vi "Process.vi"(8 "error in (no error)":errorcluster, 9 "New polarization":dbl, 10 "New eventnum":i64, 11 "Automation in":refnum<class "NMR Data.lvclass">) -> (0 "error out":errorcluster, 2 "Added new data point?":bool, 3 "Automation out":refnum<class "NMR Data.lvclass">)   [LabVIEW 2019, in "NMR Data.lvclass"]
uses:
  NMR Data.lvclass
  NMR Data.lvclass/NMR Data.ctl
panel:
  out "Eventnums":i64[](array[numeric])
  out "Polarizations":dbl[](array[numeric])
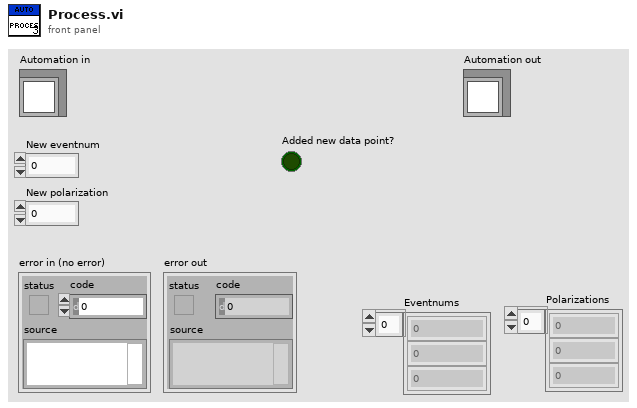
[diagram p1: front panel]
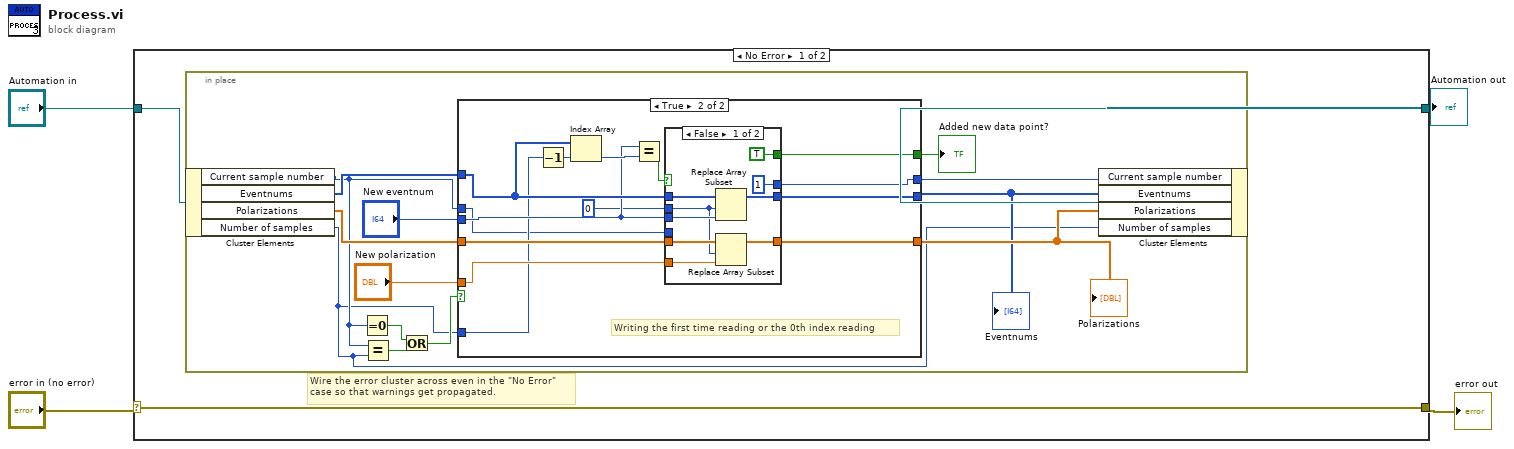
[diagram p0: block diagram]
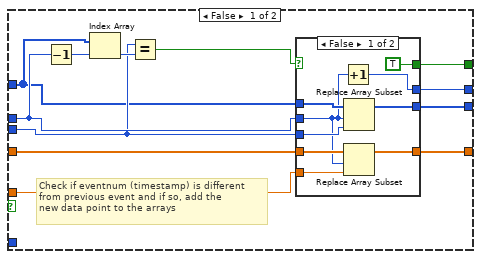
[diagram p2: hidden frame]
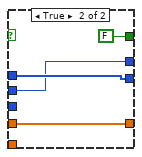
[diagram p3: hidden frame]
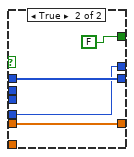
[diagram p4: hidden frame]
diagram:
  n1 = case shown="No Error" "error in (no error)" {
    selector: "error in (no error)" -> [w7 w74]
    tunnel: [w7 w74] -> w3
    tunnel: [w5 w73] -> w1
    tunnel: "Automation in" -> [w6 w73]
    frame No Error {
      # "Wire the error cluster across even in the \"No Error\"\ncase so that warnings get propagated."
      n2 = in-place {
        n3 = in-place-cluster #1(w6) -> ("Current sample number"=w12:i32, "Eventnums"=w17:i64[], "Polarizations"=w16:dbl[], "Number of samples"=w8:i32)
        n4 = Equal To 0?(x=w12) -> (x = 0?=w10:bool)
        n5 = Equal?(x=w12, y=w8) -> (x = y?=w11:bool)
        n6 = Or(x=w10, y=w11) -> (x .or. y?=w9:bool)
        n7 = case shown="True" w9 {
          tunnel: w12 -> [w29 w46]
          tunnel: [w21 w49] -> w13
          tunnel: "New eventnum" -> [w27 w52]
          tunnel: w17 -> [w25 w53]
          tunnel: w16 -> [w28 w59]
          tunnel: "New polarization" -> [w26 w58]
          tunnel: [w22 w57] -> w14
          tunnel: [w23 w56] -> w15
          tunnel: [w24 w47] -> w18
          tunnel: w8 -> [_ w48]
          frame False {
            # "Check if eventnum (timestamp) is different\nfrom previous event and if so, add the\nnew data point to the arrays"
            n8 = Decrement(x=w29) -> (x-1=w30:i32)
            n9 = Index Array(array=w25, index=w30) -> (element=w31:i64)
            n10 = Equal?(x=w27, y=w31) -> (x = y?=w32:bool)
            n11 = case shown="False" w32 {
              tunnel: [w34 w43] -> w21
              tunnel: w25 -> [w41 w44]
              tunnel: w27 -> [w40 _]
              tunnel: w29 -> [w35 w43]
              tunnel: [w39 w44] -> w22
              tunnel: w26 -> [w38 _]
              tunnel: w28 -> [w37 w45]
              tunnel: [w36 w45] -> w23
              tunnel: [TRUE FALSE] -> w24
              frame False {
                n12 = Increment(x=w35) -> (x+1=w34:i32)
                n13 = Replace Array Subset(array=w41, new element=w40, index=w35) -> (w39:i64[])
                n14 = Replace Array Subset(array=w37, new element=w38, index=w35) -> (w36:dbl[])
              }
              frame True {
              }
            }
          }
          frame True {
            # "Writing the first time reading or the 0th index reading"
            n15 = Decrement(x=w48) -> (x-1=w54:i32)
            n16 = Index Array(array=w53, index=w54) -> (element=w55:i64)
            n17 = Equal?(x=w52, y=w55) -> (x = y?=w51:bool)
            n18 = case shown="False" w51 {
              tunnel: 0 ("Current sample number") -> [w62 _]
              tunnel: w59 -> [w68 w71]
              tunnel: w58 -> [w67 _]
              tunnel: [w66 w72] -> w57
              tunnel: [w65 w71] -> w56
              tunnel: w53 -> [w64 w72]
              tunnel: w52 -> [w63 _]
              tunnel: [1 ("Current sample number") w70] -> w49
              tunnel: w46 -> [_ w70]
              tunnel: [TRUE FALSE] -> w47
              frame False {
                n19 = Replace Array Subset(array=w64, new element=w63, index=w62) -> (w66:i64[])
                n20 = Replace Array Subset(array=w68, new element=w67, index=w62) -> (w65:dbl[])
              }
              frame True {
              }
            }
          }
        }
        "Added new data point?" <- w18
        "Polarizations" <- w15
        "Eventnums" <- w14
        n21 = in-place-cluster #1("Current sample number"=w13, "Eventnums"=w14, "Polarizations"=w15, "Number of samples"=w8) -> (w5:refnum<class "NMR Data.lvclass">)
      }
    }
    frame Error {
    }
  }
  "error out" <- w3
  "Automation out" <- w1
